vi "Loop_Overloard.vi"() -> ()   [LabVIEW 2017, in "Rotation_Overloard.lvlib"]
uses:
  Rotation_Overloard.lvlib
  _SHARE ALL/Global Share All/Global_STOP.vi
  ENUM_Overloard_Action.ctl
  ENUM_Overloard_State.ctl
  Arm/ENUM_SM_Rotate_Positions.ctl
  Arm/Arm.lvlib
  Arm/CLUSTER_CMD_SM_Lift_Rotate.ctl
  Claw Rotation/ENUM_SM_Rotate_Positions.ctl
  Claw Rotation/Claw_Rotation.lvlib
  Claw Rotation/CLUSTER_CMD_SM_Lift_Rotate.ctl
  Lift/ENUM_SM_Rotate_Positions.ctl
  Lift/Lift.lvlib
  Lift/CLUSTER_CMD_SM_Lift_Rotate.ctl
  Arm/Global_CMD.vi
  Claw Rotation/Global_CMD.vi
  Lift/Global_CMD.vi
  ENUM_Rotation_Positon.ctl
  CLUSTER_Rotation_CMD.ctl
  Global_CMD.vi
  Arm/ENUM_SM_State.ctl
  Claw Rotation/ENUM_SM_State.ctl
  Lift/ENUM_SM_State.ctl
  Arm/Global_SM Write_Data Out.vi
  Claw Rotation/Global_SM Write_Data Out.vi
  Lift/Global_SM Write_Data Out.vi
panel:
  out "Input DBL Data":dbl
  out "Output Bool Data":bool
  out "Output DBL Data":dbl
  out "OutputI INT Data":i32
  out "Cycle Time (S)":dbl format="%.3g"
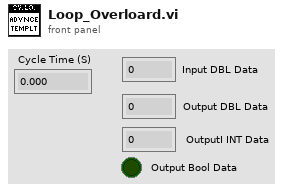
[diagram p1: front panel]
types:
  T1 = typedef "Lift.lvlib/ENUM_SM_State.ctl" = enum16{"Startup", "Idle", "Manual", "Position - Moving", "Position - Holding", "Shutdown"}
  T2 = typedef "Claw_Rotation.lvlib/ENUM_SM_State.ctl" = enum16{"Startup", "Idle", "Manual", "Position - Moving", "Position - Holding", "Shutdown"}
  T3 = typedef "Arm.lvlib/ENUM_SM_State.ctl" = enum16{"Startup", "Idle", "Manual", "Position - Moving", "Position - Holding", "Shutdown"}
  T4 = typedef "Rotation_Overloard.lvlib/CLUSTER_Rotation_CMD.ctl" = cluster{"Rotation Positon":T5, "Enable Lift":bool}
  T5 = typedef "Rotation_Overloard.lvlib/ENUM_Rotation_Positon.ctl" = enum16{"Starting", "Pickup", "Exchange", "Switch", "Scale", "Climb", "Manual"}
  T6 = typedef "Lift.lvlib/CLUSTER_CMD_SM_Lift_Rotate.ctl" = cluster{"Enable System":bool, "Rotate Position":T7, "Manual Velocity":dbl, "Manual Mode":bool}
  T7 = typedef "Lift.lvlib/ENUM_SM_Rotate_Positions.ctl" = enum16{"Starting: 0"}
  T8 = typedef "Claw_Rotation.lvlib/CLUSTER_CMD_SM_Lift_Rotate.ctl" = cluster{"Enable System":bool, "Rotate Position":T9, "Manual Velocity":dbl, "Manual Mode":bool}
  T9 = typedef "Claw_Rotation.lvlib/ENUM_SM_Rotate_Positions.ctl" = enum16{"Starting: 0"}
  T10 = typedef "Arm.lvlib/CLUSTER_CMD_SM_Lift_Rotate.ctl" = cluster{"Enable System":bool, "Rotate Position":T11, "Manual Velocity":dbl, "Manual Mode":bool}
  T11 = typedef "Arm.lvlib/ENUM_SM_Rotate_Positions.ctl" = enum16{"Starting: 0"}
  T12 = typedef "Rotation_Overloard.lvlib/ENUM_Overloard_State.ctl" = enum16{"Startup", "Idle", "Neutral Position", "Pickup Position", "Exchange Position", "Switch Position", "Scale Position", "Climb Position", "Shutdown"}
  T13 = typedef "Rotation_Overloard.lvlib/ENUM_Overloard_Action.ctl" = enum16{"No Action", "Reset Time", "Reset All", "Action A", "Action B"}
  T14 = cluster{"State":T12, "Previous State":T12, "Current Time":timestamp, "Previous Time":timestamp, "Start Time":timestamp, "Target Time (ms)":u32, "Cycle Time(S)":dbl, "Arm CMD":T10, "Claw Rotation CMD":T8, "Lift CMD":T6, "Rotation CMD":T4, "Arm State":T3, "Claw Rotation State":T2, "Lift State":T1}
  T15 = typedef "Rotation_Overloard.lvlib/ENUM_Auto_State.ctl" = enum16{"Startup", "Idle", "Auto Step 1", "Auto Step 2", "Shutdown"}
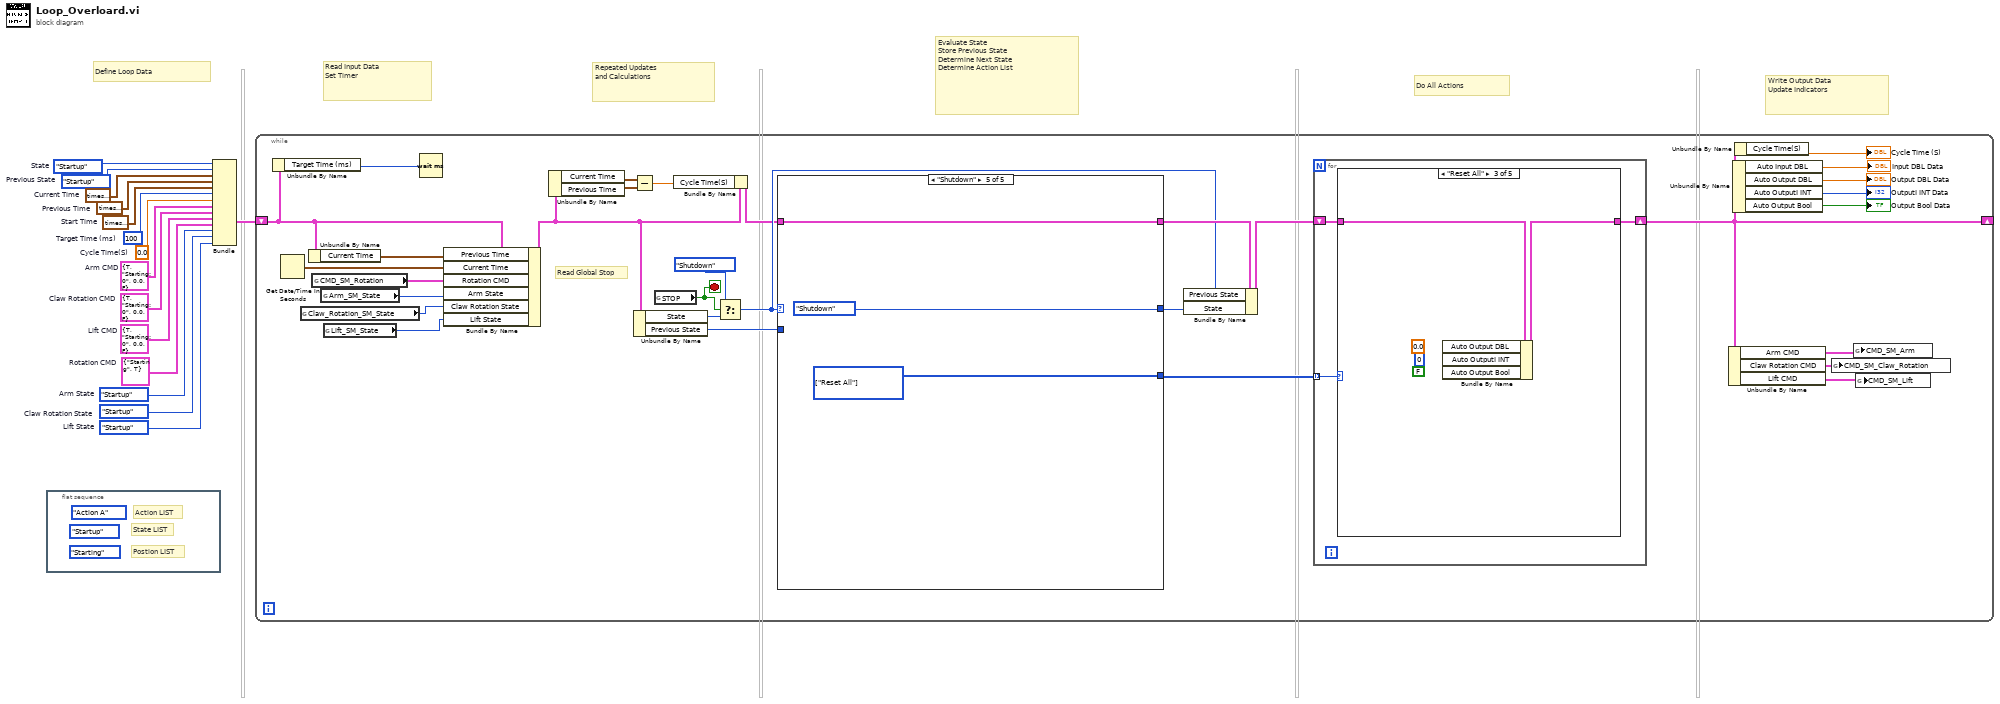
[diagram p0: block diagram]
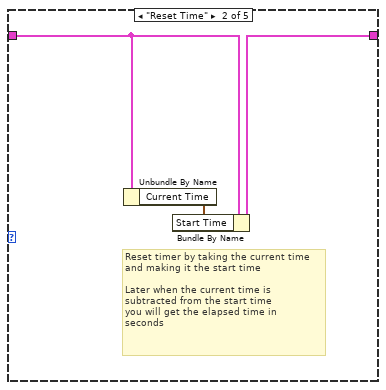
[diagram p3: hidden frame]
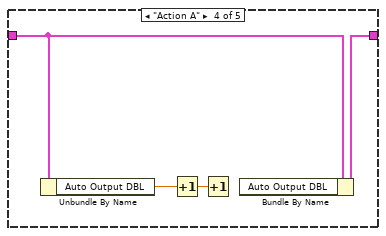
[diagram p4: hidden frame]
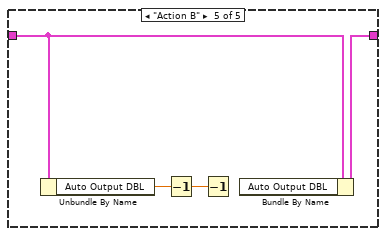
[diagram p5: hidden frame]
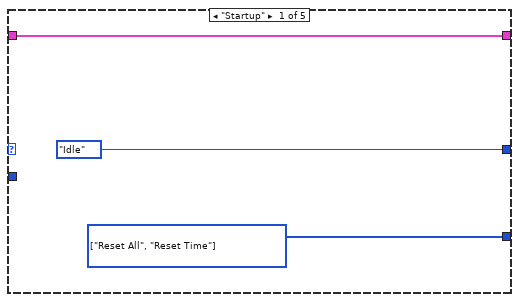
[diagram p6: hidden frame]
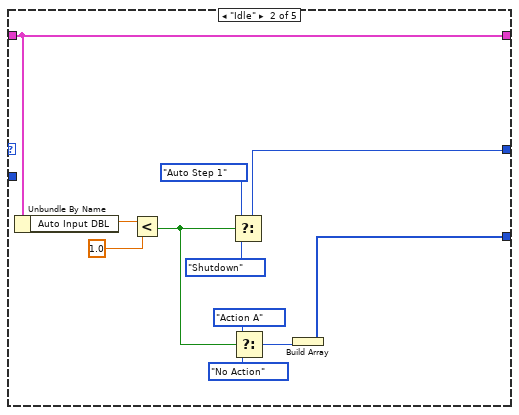
[diagram p7: hidden frame]
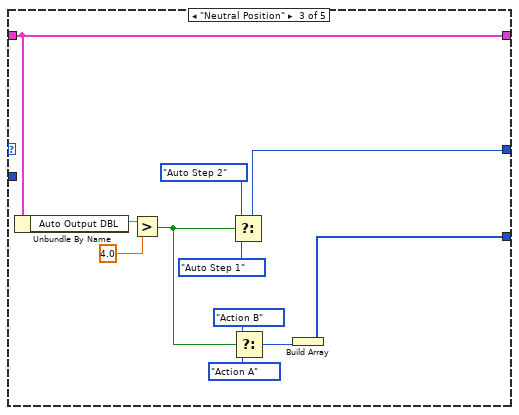
[diagram p8: hidden frame]
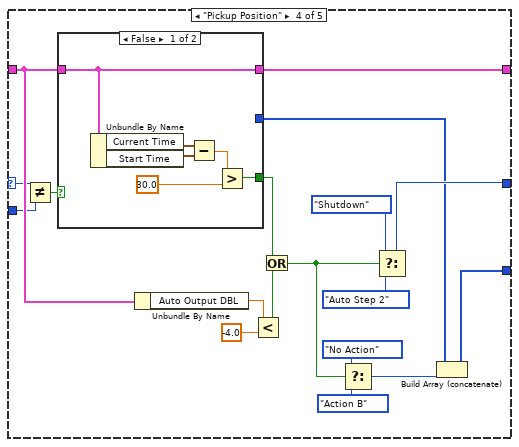
[diagram p9: hidden frame]
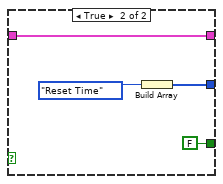
[diagram p10: hidden frame]
diagram:
  w1 = ENUM_SM_State."Startup"  # Lift State
  w2 = ENUM_SM_State."Startup"  # Claw Rotation State
  w3 = ENUM_SM_State."Startup"  # Arm State
  w4 = T4 {"Rotation Positon"=enum."Starting", "Enable Lift"=TRUE}  # Rotation CMD
  w5 = T6 {"Enable System"=TRUE, "Rotate Position"=enum."Starting: 0", "Manual Velocity"=0.0, "Manual Mode"=FALSE}  # Lift CMD
  w6 = T8 {"Enable System"=TRUE, "Rotate Position"=enum."Starting: 0", "Manual Velocity"=0.0, "Manual Mode"=FALSE}  # Claw Rotation CMD
  w7 = T10 {"Enable System"=TRUE, "Rotate Position"=enum."Starting: 0", "Manual Velocity"=0.0, "Manual Mode"=FALSE}  # Arm CMD
  w8 = 0.0  # Cycle Time(S)
  w9 = ENUM_Overloard_State."Startup"  # Previous State
  w10 = timestamp(0 s since 1904-01-01)  # Previous Time
  w11 = u32 100  # Target Time (ms)
  w12 = timestamp(0 s since 1904-01-01)  # Start Time
  w13 = timestamp(0 s since 1904-01-01)  # Current Time
  w14 = ENUM_Overloard_State."Startup"  # State
  # "Define Loop Data"
  # "Repeated Updates\nand Calculations"
  # "Read Input Data\nSet Timer"
  # "Evaluate State\nStore Previous State\nDetermine Next State\nDetermine Action List"
  # "Do All Actions"
  # "Write Output Data\nUpdate Indicators"
  n1 = flat-sequence {
    frame #0 {
      (unwired) ENUM_Rotation_Positon."Starting" ("Rotation Position")
      (unwired) ENUM_Overloard_State."Startup" ("State")
      (unwired) ENUM_Overloard_Action."Action A" ("Action")
      # "Postion LIST"
      # "State LIST"
      # "Action LIST"
    }
  }
  n2 = Bundle("State"=w14, "Previous State"=w9, "Current Time"=w13, "Previous Time"=w10, "Start Time"=w12, "Target Time (ms)"=w11, "Cycle Time(S)"=w8, "Arm CMD"=w7, "Claw Rotation CMD"=w6, "Lift CMD"=w5, "Rotation CMD"=w4, "Arm State"=w3, "Claw Rotation State"=w2, "Lift State"=w1) -> (w15:T14)  [unwired: 1 in]
  n3 = while {
    shift-right: [w32] -> _
    shift-left: w15 -> [w38]
    stop <- w20 stop-if-true
    # "Read Global Stop"
    n4 = Unbundle By Name(w38) -> ("Target Time (ms)"=w40:u32)
    n5 = Get Date/Time In Seconds() -> (seconds since 1Jan1904=w46:timestamp)
    n6 = global read "Global_SM Write_Data Out.vi" "Claw_Rotation_SM_State"() -> (w17:T2)
    n7 = Unbundle By Name(w38) -> ("Current Time"=w39:timestamp)
    n8 = global read "Global_CMD.vi" "CMD_SM_Rotation"() -> (w19:T4)
    n9 = global read "Global_SM Write_Data Out.vi" "Arm_SM_State"() -> (w18:T3)
    n10 = global read "Global_SM Write_Data Out.vi" "Lift_SM_State"() -> (w16:T1)
    n11 = Wait (ms)(milliseconds to wait=w40) -> ()  [unwired: 1 out]
    n12 = Bundle By Name(cluster=w38, "Previous Time"=w39, "Current Time"=w46, "Rotation CMD"=w19, "Arm State"=w18, "Claw Rotation State"=w17, "Lift State"=w16) -> (w28:T14)
    n13 = Unbundle By Name(w28) -> ("Current Time"=w29:timestamp, "Previous Time"=w30:timestamp)
    n14 = Subtract(x=w29, y=w30) -> (x-y=w26:dbl)
    n15 = Unbundle By Name(w28) -> ("State"=w41:T12, "Previous State"=w37:T12)
    n16 = global read "Global_STOP.vi" "STOP"() -> (w20:bool)
    n17 = Bundle By Name(cluster=w28, "Cycle Time(S)"=w26) -> (w27:T14)
    n18 = Select(t=ENUM_Overloard_State."Shutdown" ("State"), s=w20, f=w41) -> (s? t:f=w33:T12)
    n19 = case shown="\"Shutdown\"" w33 {
      selector: w33 -> [_ _ _ w92 _]
      tunnel: w27 -> [w66 w77 w88 w94 w119]
      tunnel: [w66 w77 w88 w93 w119] -> w44
      tunnel: [ENUM_Overloard_State."Idle" ("State") w76 w87 w106 ENUM_Overloard_State."Shutdown" ("State")] -> w43
      tunnel: [w65 w69 w80 w99 w117] -> w25
      tunnel: w37 -> [_ _ _ w91 _]
      frame "Startup" {
        w65 = T13[] [enum."Reset All", enum."Reset Time"] items=["No Action", "Reset Time", "Reset All", "Action A", "Action B"] ("Actions")
      }
      frame "Idle" {
        n20 = Unbundle By Name(w77) -> ("Auto Input DBL"=w68:dbl)
        n21 = Less?(x=w68, y=1.0) -> (x < y?=w71:bool)
        n22 = Select(t=ENUM_Auto_State."Auto Step 1" ("State"), s=w71, f=ENUM_Overloard_State."Shutdown" ("State")) -> (s? t:f=w76:u16)
        n23 = Select(t=ENUM_Overloard_Action."Action A" ("Action"), s=w71, f=ENUM_Overloard_Action."No Action" ("Action")) -> (s? t:f=w70:T13)
        n24 = Build Array(w70) -> (w69:T13[])
      }
      frame "Neutral Position" {
        n25 = Unbundle By Name(w88) -> ("Auto Output DBL"=w79:dbl)
        n26 = Greater?(x=w79, y=4.0) -> (0:w82:bool)
        n27 = Select(t=ENUM_Auto_State."Auto Step 2" ("State"), s=w82, f=ENUM_Auto_State."Auto Step 1" ("State")) -> (s? t:f=w87:T15)
        n28 = Select(t=ENUM_Overloard_Action."Action B" ("Action"), s=w82, f=ENUM_Overloard_Action."Action A" ("Action")) -> (s? t:f=w81:T13)
        n29 = Build Array(w81) -> (w80:T13[])
      }
      frame "Pickup Position" {
        n30 = Not Equal?(x=w92, y=w91) -> (x != y?=w90:bool)
        n31 = case shown="False" w90 {
          tunnel: [w112 FALSE] -> w101
          tunnel: w94 -> [w107 w115]
          tunnel: [w107 w115] -> w93
          tunnel: [_ w113] -> w89
          frame False {
            n32 = Unbundle By Name(w107) -> ("Current Time"=w110:timestamp, "Start Time"=w109:timestamp)
            n33 = Subtract(x=w110, y=w109) -> (x-y=w108:dbl)
            n34 = Greater?(x=w108, y=30.0) -> (0:w112:bool)
          }
          frame True {
            n35 = Build Array(ENUM_Overloard_Action."Reset Time" ("Action")) -> (w113:T13[])
          }
        }
        n36 = Unbundle By Name(w94) -> ("Auto Output DBL"=w97:dbl)
        n37 = Less?(x=w97, y=-4.0) -> (x < y?=w95:bool)
        n38 = Or(x=w101, y=w95) -> (x .or. y?=w98:bool)
        n39 = Select(t=ENUM_Overloard_Action."No Action" ("Action"), s=w98, f=ENUM_Overloard_Action."Action B" ("Action")) -> (s? t:f=w100:T13)
        n40 = Select(t=ENUM_Overloard_State."Shutdown" ("State"), s=w98, f=ENUM_Auto_State."Auto Step 2" ("State")) -> (s? t:f=w106:u16)
        n41 = Build Array (concatenate)(w89, w100) -> (w99:T13[])
      }
      frame "Shutdown" {
        w117 = T13[] [enum."Reset All"] items=["No Action", "Reset Time", "Reset All", "Action A", "Action B"] ("Actions")
      }
    }
    n42 = Bundle By Name(cluster=w44, "Previous State"=w33, "State"=w43) -> (w45:T14)
    n43 = for {
      tunnel: w25 -> [w49] mode=indexing
      shift-right: [w48] -> w32
      shift-left: w45 -> [w47]
      n44 = case shown="\"Reset All\"" w49 {
        tunnel: w47 -> [w50 w53 w55 w58 w62]
        tunnel: [w50 w52 w54 w57 w61] -> w48
        frame "No Action" {
        }
        frame "Reset Time" {
          # "Reset timer by taking the current time\nand making it the start time\n\nLater when the current time is \nsubtracted from the start time\nyou will get the elapsed time in \nseconds"
          n45 = Unbundle By Name(w53) -> ("Current Time"=w51:timestamp)
          n46 = Bundle By Name(cluster=w53, "Start Time"=w51) -> (w52:T14)
        }
        frame "Reset All" {
          (unwired) FALSE ("Output Bool")
          (unwired) 0 ("OutputI INT")
          (unwired) 0.0 ("FG Write Value")
          n47 = Bundle By Name(cluster=w55) -> (w54:T14)  [unwired: 3 in]
        }
        frame "Action A" {
          n48 = Unbundle By Name(w58) -> ("Auto Output DBL"=w59:dbl)
          n49 = Increment(x=w59) -> (x+1=w56:dbl)
          n50 = Increment(x=w56) -> ()  [unwired: 1 out]
          n51 = Bundle By Name(cluster=w58) -> (w57:T14)  [unwired: 1 in]
        }
        frame "Action B" {
          n52 = Unbundle By Name(w62) -> ("Auto Output DBL"=w63:dbl)
          n53 = Decrement(x=w63) -> (x-1=w60:dbl)
          n54 = Decrement(x=w60) -> ()  [unwired: 1 out]
          n55 = Bundle By Name(cluster=w62) -> (w61:T14)  [unwired: 1 in]
        }
      }
    }
    n56 = Unbundle By Name(w32) -> ("Arm CMD"=w23:T10, "Claw Rotation CMD"=w22:T8, "Lift CMD"=w21:T6)
    n57 = Unbundle By Name(w32) -> ("Auto Input DBL"=→"Input DBL Data":dbl, "Auto Output DBL"=→"Output DBL Data":dbl, "Auto OutputI INT"=→"OutputI INT Data":i32, "Auto Output Bool"=→"Output Bool Data":bool)
    n58 = Unbundle By Name(w32) -> ("Cycle Time(S)"=→"Cycle Time (S)":dbl)
    n59 = global write "Global_CMD.vi" "CMD_SM_Claw_Rotation"(w22) -> ()
    n60 = global write "Global_CMD.vi" "CMD_SM_Arm"(w23) -> ()
    n61 = global write "Global_CMD.vi" "CMD_SM_Lift"(w21) -> ()
  }
